vi "CSV Configuration Reader.vi"(10 "Section":string, 11 "All CSV Configurations":string[][](array[string])) -> (2 "Section Exists?":bool, 3 "Extracted Configurations":string[][](array[string]))   [LabVIEW 2023]
uses:
  <vilib>/Utility/error.llb/Trim Whitespace One-Sided.vi
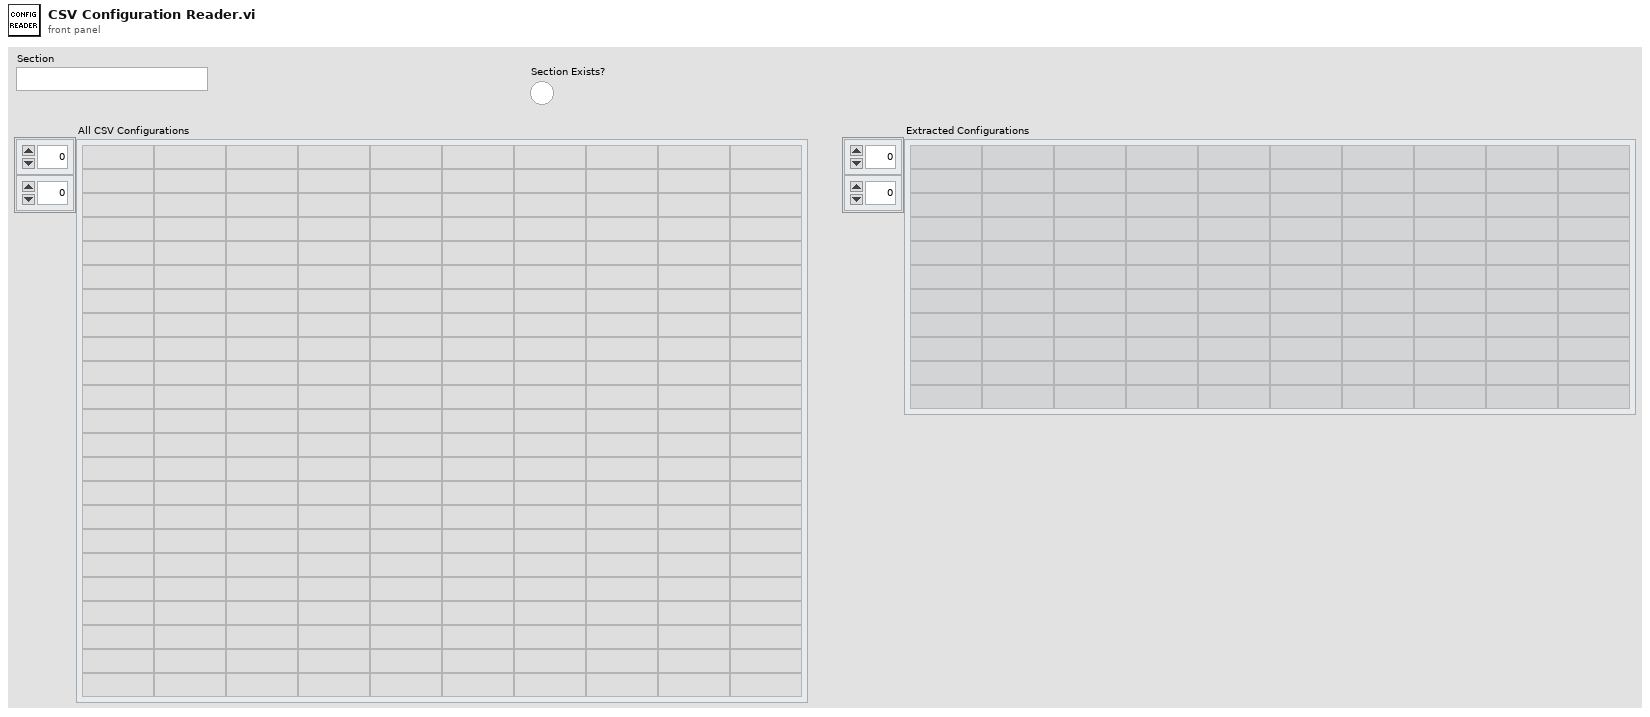
[diagram p1: front panel]
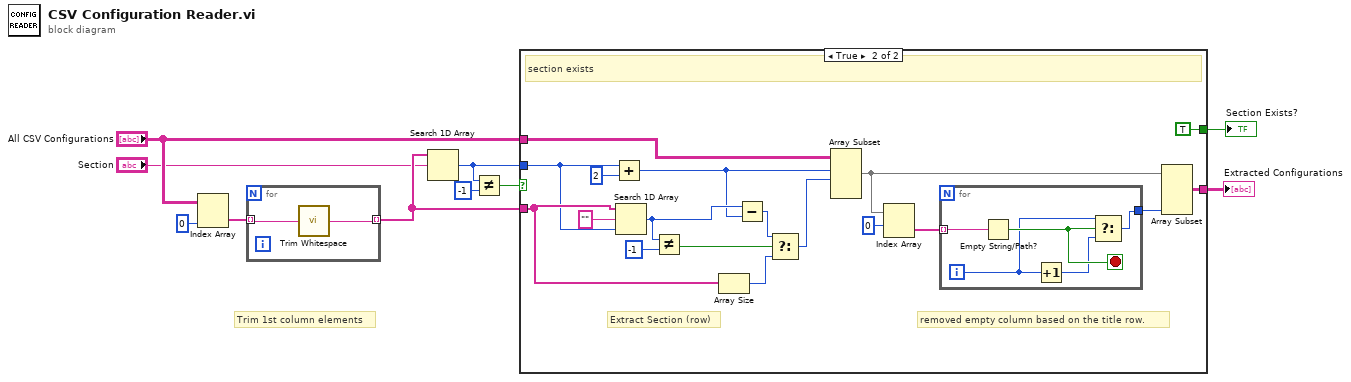
[diagram p0: block diagram]
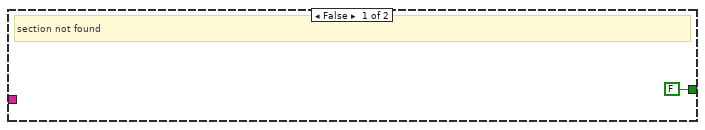
[diagram p2: hidden frame]
diagram:
  # "Trim 1st column elements"
  n1 = Index Array(array="All CSV Configurations", index (col)=0 ("disabled index (col)")) -> (element=w7:string[])  [unwired: 1 in]
  n2 = for {
    tunnel: w7 -> [w12] mode=indexing
    tunnel: [w11] -> w10 mode=indexing
    n3 = call <vilib>:"Trim Whitespace.vi"("string"=w12) -> ("trimmed string"=w11:string)  [unwired: 1 in]
  }
  n4 = Search 1D Array(1D array=w10, element="Section") -> (index of element=w4:i32)  [unwired: 1 in]
  n5 = Not Equal?(x=w4, y=-1) -> (x != y?=w2:bool)
  n6 = case shown="True" w2 {
    tunnel: w10 -> [_ w30]
    tunnel: "All CSV Configurations" -> [_ w23]
    tunnel: w4 -> [_ w22]
    tunnel: [_ w17] -> w5
    tunnel: [FALSE TRUE] -> w1
    frame False {
      # "section not found"
    }
    frame True {
      # "removed empty column based on the title row."
      # "Extract Section (row)"
      # "section exists"
      n7 = Add(x=w22, y=2) -> (x+y=w24:i32)
      n8 = Search 1D Array(1D array=w30, element="", start index (0)=w22) -> (index of element=w26:i32)
      n9 = Not Equal?(x=w26, y=-1) -> (x != y?=w28:bool)
      n10 = Array Size(array=w30) -> (size(s)=w31:i32)
      n11 = Subtract(x=w26, y=w24) -> (x-y=w27:i32)
      n12 = Select(t=w27, s=w28, f=w31) -> (s? t:f=w29:i32)
      n13 = Array Subset(array=w23, index (row)=w24, length (row)=w29) -> (w16:string[][])  [unwired: 2 in]
      n14 = Index Array(array=w16, index (row)=0) -> (element=w18:string[])  [unwired: 1 in]
      n15 = for {
        tunnel: w18 -> [w36] mode=indexing
        tunnel: [w35] -> w15
        i -> [w33]
        stop <- w34 stop-if-true
        n16 = Empty String/Path?(string/path=w36) -> (empty?=w34:bool)
        n17 = Increment(x=w33) -> (x+1=w32:i32)
        n18 = Select(t=w33, s=w34, f=w32) -> (s? t:f=w35:i32)
      }
      n19 = Array Subset(array=w16, length (col)=w15) -> (w17:string[][])  [unwired: 3 in]
    }
  }
  "Extracted Configurations" <- w5
  "Section Exists?" <- w1
